vi "connect.vi"(6 "timeout ms (10000)":i32=10000, 8 "error in":errorcluster, 11 "connection client in":refnum<class "connection client.lvclass">) -> (0 "error out":errorcluster, 1 "valid?":bool, 2 "connection handler":refnum<class "connection maintainer.lvclass">, 3 "connection client out":refnum<class "connection client.lvclass">)   [LabVIEW 2015, in "connection client.lvclass"]
uses:
  connection client.lvclass
  connection/connection maintainer.lvclass
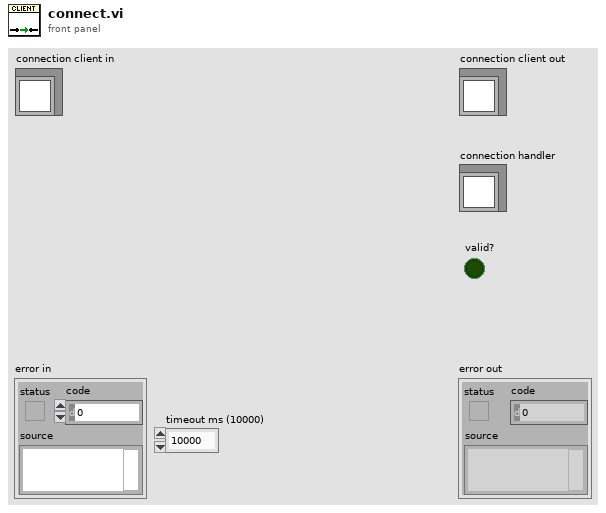
[diagram p1: front panel]
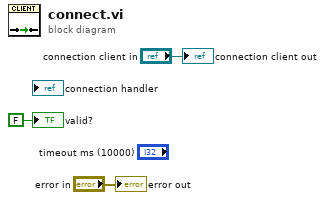
[diagram p0: block diagram]
diagram:
  "error out" <- "error in"
  "connection client out" <- "connection client in"
  "valid?" <- FALSE ("valid?")
